vi "Get Active Statement Function.vi"(0 "Statement in":refnum<class "DMM.lvclass">=refnum, 11 "error in (no error)":errorcluster) -> (4 "Statement out":refnum<class "DMM.lvclass">, 6 "Function List":T1, 15 "error out":errorcluster)   [LabVIEW 2019, in "DMM.lvclass"]
uses:
  DMM.lvclass
  source code/LSL components/functions/functionsbase/functionbase.lvclass
  Function List.ctl
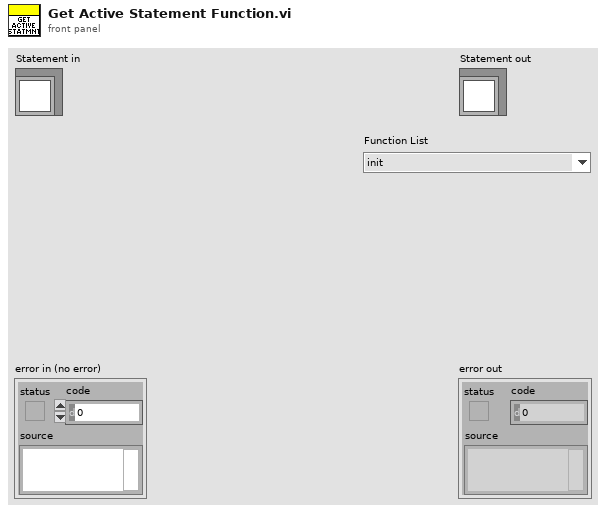
[diagram p1: front panel]
types:
  T1 = typedef "DMM.lvclass/Function List.ctl" = enum16{"init", "measure", "close", "close all"}
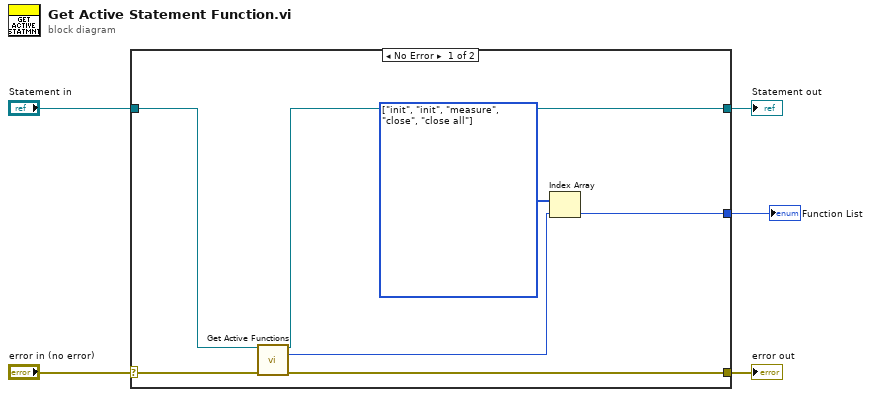
[diagram p0: block diagram]
diagram:
  n1 = case shown="No Error" "error in (no error)" {
    selector: "error in (no error)" -> [w12 w14]
    tunnel: [w11 w14] -> w4
    tunnel: [w9 w13] -> w2
    tunnel: "Statement in" -> [w10 w13]
    tunnel: [w6 _] -> w1
    frame No Error {
      w7 = T1[] [enum."init", enum."init", enum."measure", enum."close", enum."close all"] items=["init", "measure", "close", "close all"]
      n2 = call "Get Active Functions.vi"("functionbase in"=w10, "error in (no error)"=w12) -> ("functionbase out"=w9:refnum<class "functionbase.lvclass">, "Syntax Index"=w8:i32, "error out"=w11:errorcluster)  [unwired: 11 in]
      n3 = Index Array(array=w7, index=w8) -> (element=w6:T1)
    }
    frame Error {
    }
  }
  "error out" <- w4
  "Statement out" <- w2
  "Function List" <- w1
